vi "ABB secs to hr-min-sec.vi"(9 "round off secs":bool, 10 "Precision":i16, 11 "Seconds":dbl) -> (3 "hr:min:secs":string)   [LabVIEW 2017]
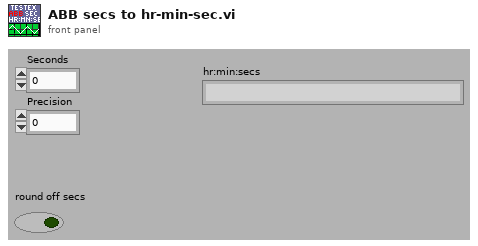
[diagram p1: front panel]
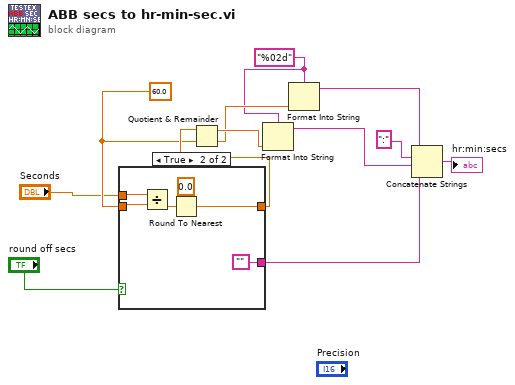
[diagram p0: block diagram]
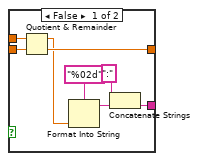
[diagram p2: hidden frame]
diagram:
  w4 = "%02d" ("format string")
  w11 = 60.0 ("y")
  n1 = case shown="True" "round off secs" {
    tunnel: "Seconds" -> [w20 w25]
    tunnel: [w19 w22] -> w12
    tunnel: w11 -> [w18 w24]
    tunnel: [w14 ""] -> w1
    frame False {
      n2 = Quotient & Remainder(x=w20, y=w18) -> (x-y*floor(x/y)=w16:dbl, floor(x/y)=w19:dbl)
      n3 = Format Into String(format string="%02d", w16) -> (resulting string=w15:string)  [unwired: 2 in, 1 out]
      n4 = Concatenate Strings(":", w15) -> (w14:string)
    }
    frame True {
      (unwired) 0.0
      n5 = Divide(x=w25, y=w24) -> (x/y=w23:dbl)
      n6 = Round To Nearest(number=w23) -> (nearest integer value=w22:dbl)
    }
  }
  n7 = Quotient & Remainder(x=w12, y=w11) -> (x-y*floor(x/y)=w8:dbl, floor(x/y)=w5:dbl)
  n8 = Format Into String(format string=w4, w8) -> (resulting string=w7:string)  [unwired: 2 in, 1 out]
  n9 = Format Into String(format string=w4, w5) -> (resulting string=w6:string)  [unwired: 2 in, 1 out]
  n10 = Concatenate Strings(w6, ":", w7, w1) -> (→"hr:min:secs":string)
